vi "I8.vi"(4 "Value":i8) -> (1 "Constant":refnum<class "Abs_I8 Integer.lvclass">)   [LabVIEW 2021, in "Const_I8.lvclass"]
uses:
  Const_I8.lvclass
  Abs_Types/I8 Integer/Abs_I8 Integer.lvclass
  C:/Program Files (x86)/National Instruments/LabVIEW 2021/vi.lib/TSA/Abstract Data Classes/Abs_Types/I8 Integer/Abs_I8 Integer.lvclass
  Const_I8.lvclass/Const_I8.ctl
  Properties/Write Value.vi
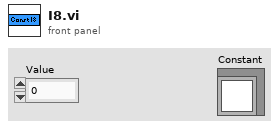
[diagram p1: front panel]
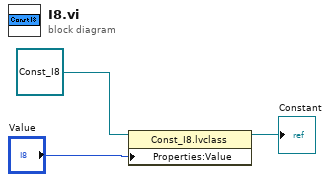
[diagram p0: block diagram]
diagram:
  n1 = property class="Const_I8.lvclass"(reference=refnum<class "Const_I8.lvclass"> refnum ("Constants.lvlib:Numeric.lvclass"), "Properties:Value"="Value") -> (reference out=→"Constant":refnum<class "Const_I8.lvclass">)  [unwired: 1 in, 1 out]
